vi "GEN_String to String Array.vi"(10 "String in":string) -> (2 "String Array out":string[](array[string]))   [LabVIEW 2016]
panel:
  in  "分隔符(,)":string=","
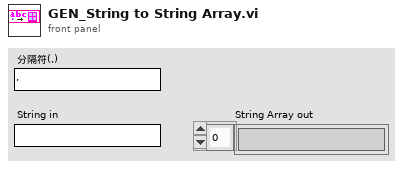
[diagram p1: front panel]
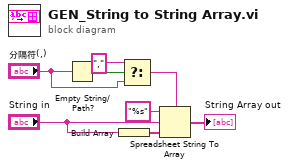
[diagram p0: block diagram]
diagram:
  n1 = Empty String/Path?(string/path="分隔符(,)") -> (empty?=w4:bool)
  n2 = Build Array("String in") -> (w7:string[])
  n3 = Select(t="," ("分隔符(,)"), s=w4, f="分隔符(,)") -> (s? t:f=w1:string)
  n4 = Spreadsheet String To Array(delimiter (Tab)=w1, format string="%s" ("格式字符串"), spreadsheet string="String in", array type (2D Dbl)=w7) -> (array=→"String Array out":string[])
